vi "4-8 tlc_Cue Module.vi"(5 "채널의 개수":cluster{"행":i32, "열":i32}, 6 "명령":T3, 7 "에러 입력(에러 없음)":errorcluster, 8 "큐 입력":T1 {"채널열"."강도" min=0.0 max=100.0 step=1.0 format="%#.0f"}, 9 "스왑 인덱스":i32 min=0, 10 "큐 인덱스":i32 min=0) -> (0 "에러 출력":errorcluster, 1 "큐 출력":T1 {"채널열"."강도" min=0.0 max=100.0 step=1.0 format="%#.0f"}, 2 "큐의 개수":i32)   [LabVIEW 2018]
doc: "Controls access to the Cue data."
panel:
  # "출력"
  # "입력"
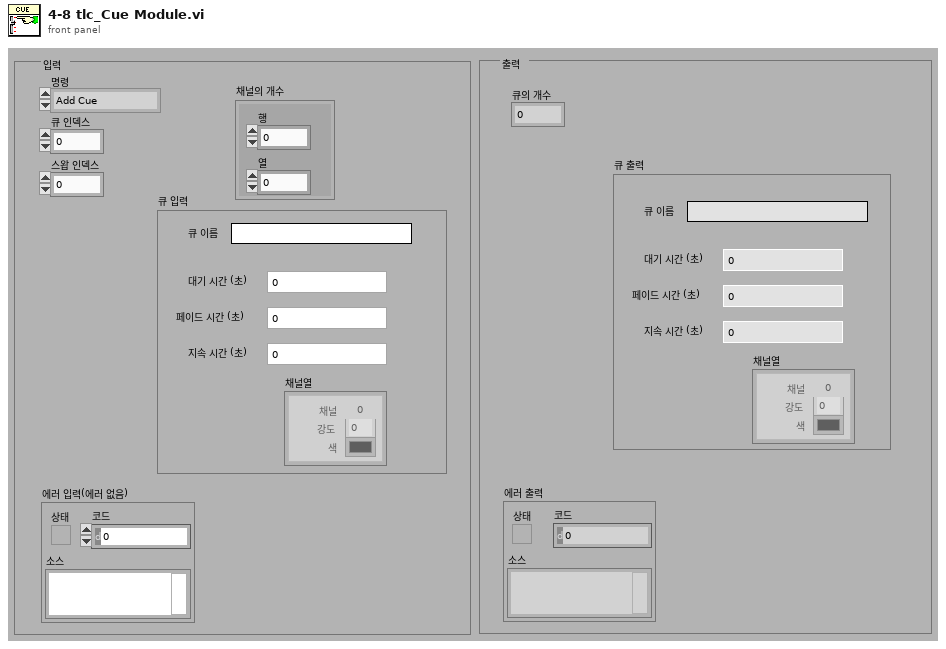
[diagram p1: front panel]
types:
  T1 = typedef "tlc_Cue_Information.ctl" = cluster{"큐 이름":string, "대기 시간 (초)":u32, "페이드 시간 (초)":u32, "지속 시간 (초)":u32, "채널열":T2[][]}
  T2 = typedef "channel.ctl" = cluster{"강도":dbl, " 색":u32, "채널":i32}
  T3 = typedef "tlc_Cue_Information Command.ctl" = enum16{"Add Cue", "Delete Cue", "Get Cue Values", "Set Cue Values", "Swap", "Get Number of Cues", "Initialize", "Get Empty Cue"}
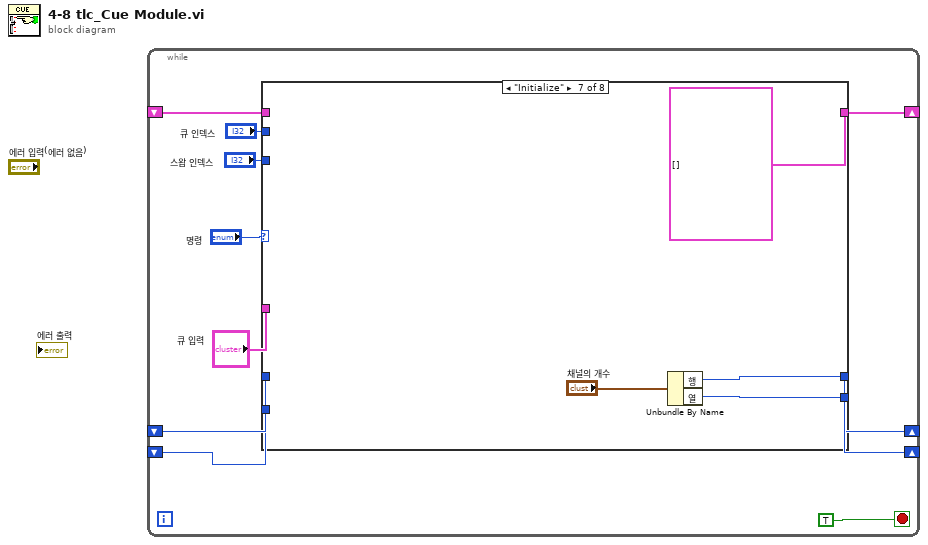
[diagram p0: block diagram]
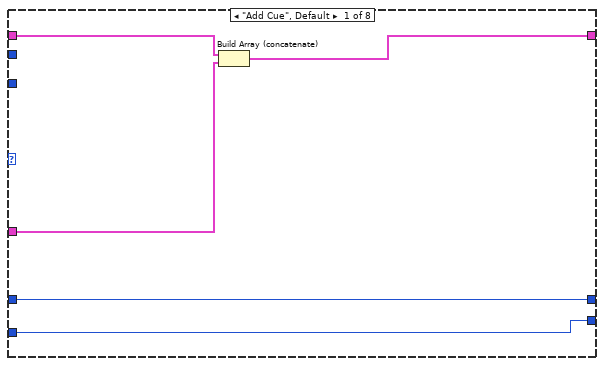
[diagram p2: hidden frame]
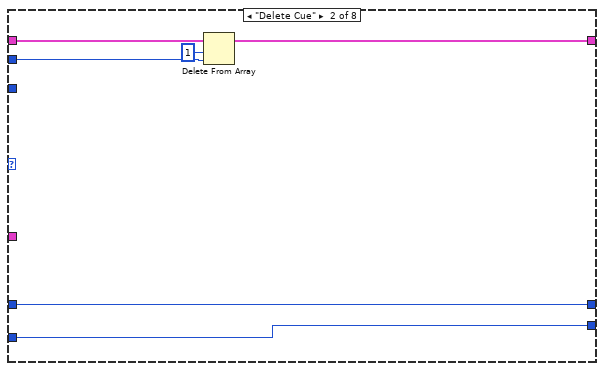
[diagram p3: hidden frame]
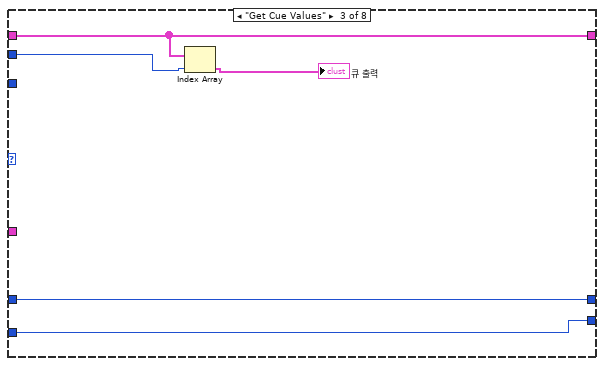
[diagram p4: hidden frame]
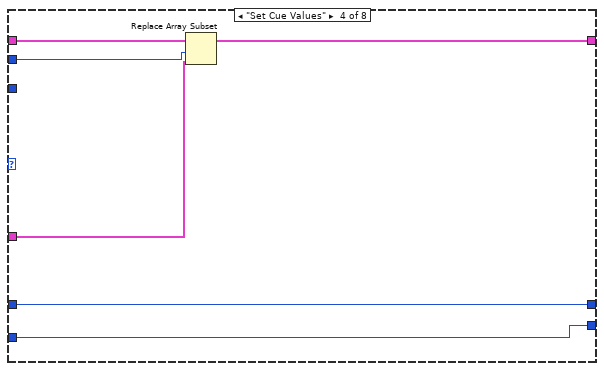
[diagram p5: hidden frame]
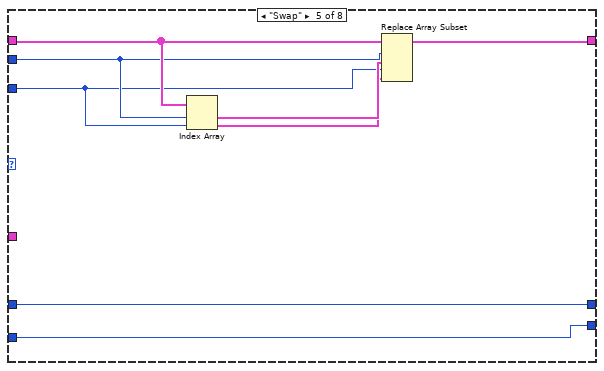
[diagram p6: hidden frame]
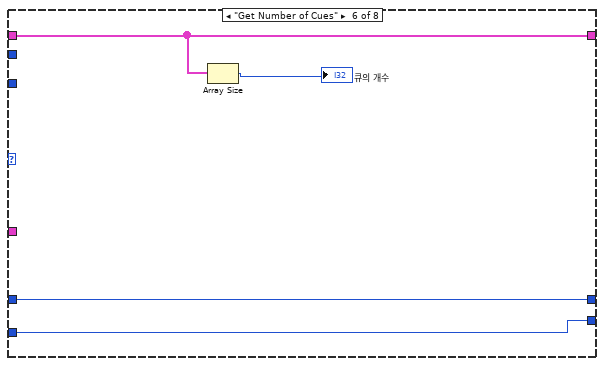
[diagram p7: hidden frame]
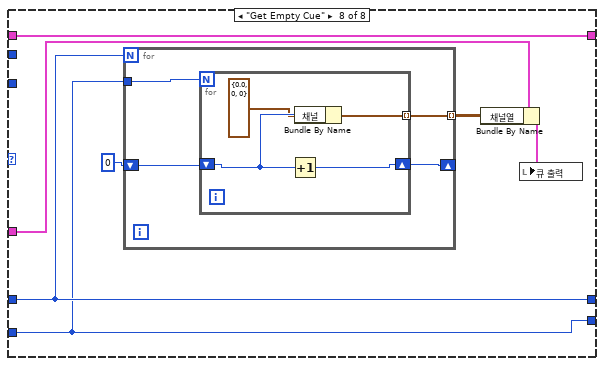
[diagram p8: hidden frame]
diagram:
  n1 = while {
    shift-right: [w1] -> _
    shift-left: _ -> [w11]
    shift-right: [w10] -> _
    shift-left: _ -> [w9]
    shift-right: [w4] -> _
    shift-left: _ -> [w7]
    stop <- TRUE stop-if-true
    n2 = case shown="\"Initialize\"" "명령" {
      tunnel: w11 -> [w13 w22 w24 w29 w35 w43 _ w55]
      tunnel: [w12 w21 w23 w28 w34 w42 w46 w54] -> w10
      tunnel: w9 -> [w12 w21 w23 w28 w34 w42 _ w54]
      tunnel: w7 -> [w14 w20 w27 w33 w40 w45 _ w56]
      tunnel: "큐 입력" -> [w16 _ _ w31 _ _ _ w52]
      tunnel: [w15 w19 w27 w32 w41 w45 T1[] [] w56] -> w4
      tunnel: "큐 인덱스" -> [_ w17 w26 w30 w37 _ _ _]
      tunnel: "스왑 인덱스" -> [_ _ _ _ w36 _ _ _]
      tunnel: [w13 w22 w24 w29 w35 w43 w47 w55] -> w1
      frame "Add Cue", Default {
        n3 = Build Array (concatenate)(w14, w16) -> (w15:T1[])
      }
      frame "Delete Cue" {
        n4 = Delete From Array(array=w20, length=1 ("길이"), index=w17) -> (array with subset deleted=w19:T1[])  [unwired: 1 out]
      }
      frame "Get Cue Values" {
        n5 = Index Array(array=w27, index=w26) -> (element=→"큐 출력":T1)
      }
      frame "Set Cue Values" {
        n6 = Replace Array Subset(array=w33, new element=w31, index=w30) -> (w32:T1[])
      }
      frame "Swap" {
        n7 = Index Array(array=w40, index #1=w37, index #2=w36) -> (element #1=w39:T1, element #2=w38:T1)
        n8 = Replace Array Subset(array=w40, new element #1=w39, index #1=w37, new element #2=w38, index #2=w36) -> (w41:T1[])
      }
      frame "Get Number of Cues" {
        n9 = Array Size(array=w45) -> (size(s)=→"큐의 개수":i32)
      }
      frame "Initialize" {
        n10 = Unbundle By Name("채널의 개수") -> ("행"=w47:i32, "열"=w46:i32)
      }
      frame "Get Empty Cue" {
        n11 = for {
          N: w55 -> [_]
          tunnel: w54 -> [w60]
          shift-right: [w58] -> _
          shift-left: 0 -> [w59]
          tunnel: [w57] -> w51 mode=indexing
          n12 = for {
            N: w60 -> [_]
            shift-right: [w64] -> w58
            shift-left: w59 -> [w63]
            tunnel: [w62] -> w57 mode=indexing
            n13 = Increment(x=w63) -> (x+1=w64:i32)
            n14 = Bundle By Name(cluster=T2 {"강도"=0.0, " 색"=0, "채널"=0} ("UI 채널"), "채널"=w63) -> (w62:T2)
          }
        }
        n15 = Bundle By Name(cluster=w52, "채널열"=w51) -> (w50:T1)
        n16 = local write "큐 출력"(w50) -> ()
      }
    }
  }
